vi "Baud rate Detect1.vi"(10 "DevIndex":u32, 11 "type":u16(ring)=2 items=["USB-CAN"=2, "USB-CAN2.0"=3]) -> ()   [LabVIEW 2011]
uses:
  _USB_CAN_GLOBAL_.vi
  data/VCI_CAN.dll
panel:
  in  "cancel":bool
  in  "ok":bool
  out "br":u32(ring)=8 caption="当前波特率:" items=["5k bps"=1, "10k bps"=2, "20k bps"=3, "40k bps"=4, "50k bps"=5, "80k bps"=6, "100k bps"=7, "125k bps"=8, "200k bps"=9, "250k bps"=10, "400k bps"=11, "500k bps"=12, "666k bps"=13, "800k bps"=14, "1000k bps"=15, "self define"=16]
  out "chl":u32 caption="正在侦测：" format="通道%d"
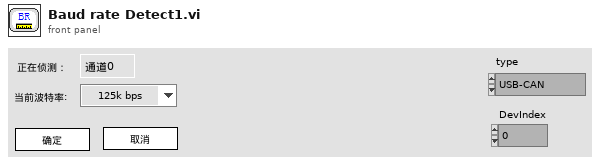
[diagram p1: front panel]
types:
  T1 = cluster{"AccCode":u32, "AccMask":u32, "Reserved":u32, "Filter":u8, "kCanBaud":u8, "Timing0":u8, "Timing1":u8, "Mode":u8}
  T2 = enum8{"Enabled", "Disabled", "Disabled and Grayed Out"}
  T3 = cluster{"ErrInterrupt":u8, "regMode":u8, "regStatus":u8, "regALCapture":u8, "regECCapture":u8, "regEWLimit":u8, "regRECounter":u8, "regTECounter":u8, "Reserved":u32}
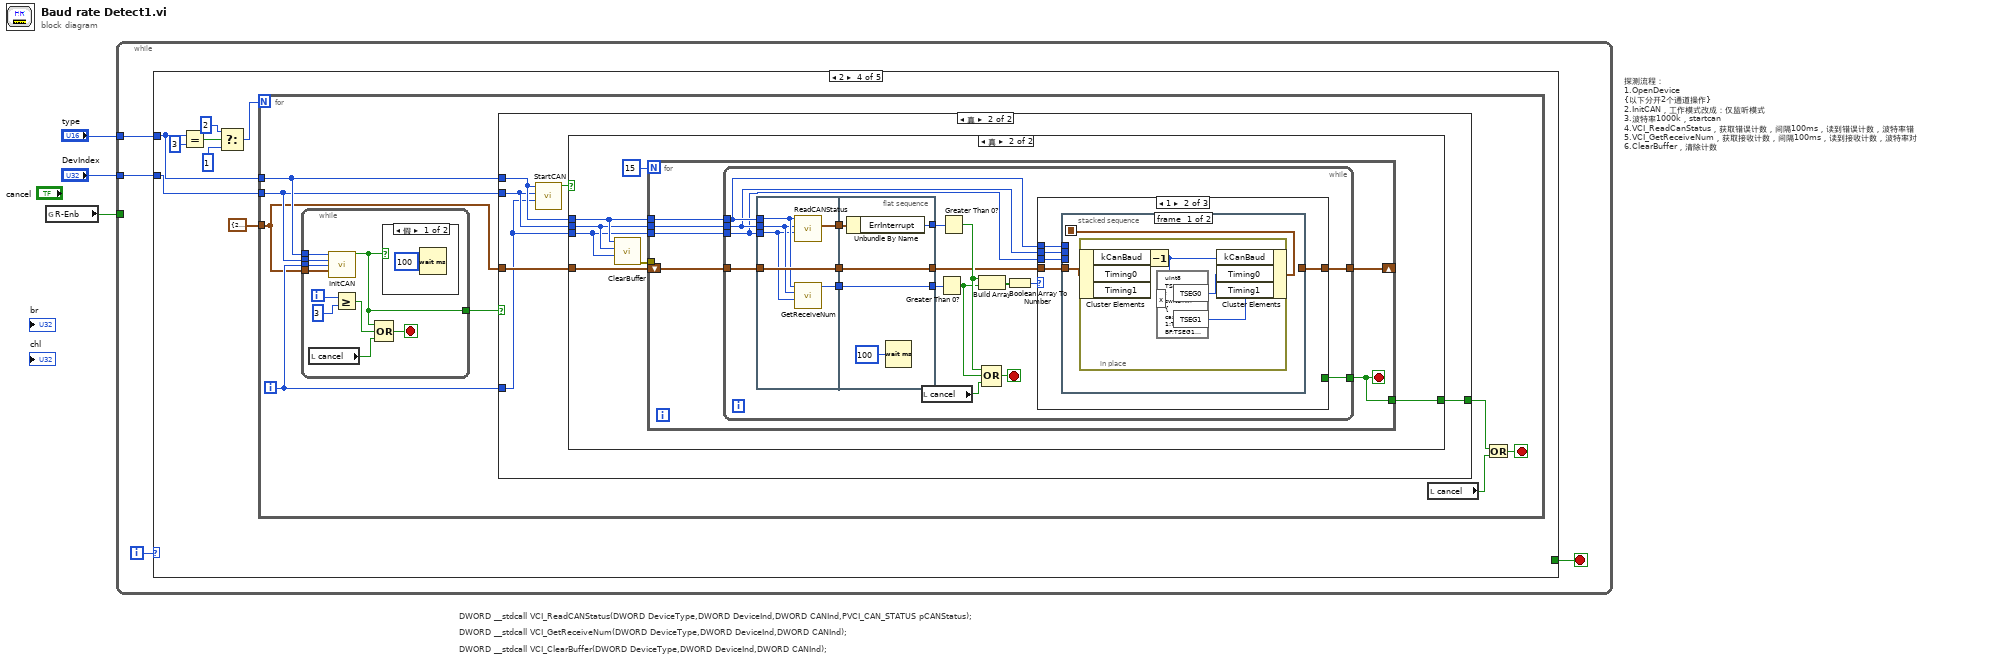
[diagram p0: block diagram]
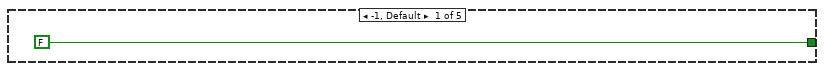
[diagram p2: hidden frame]
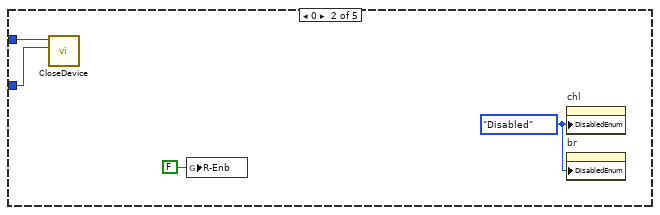
[diagram p3: hidden frame]
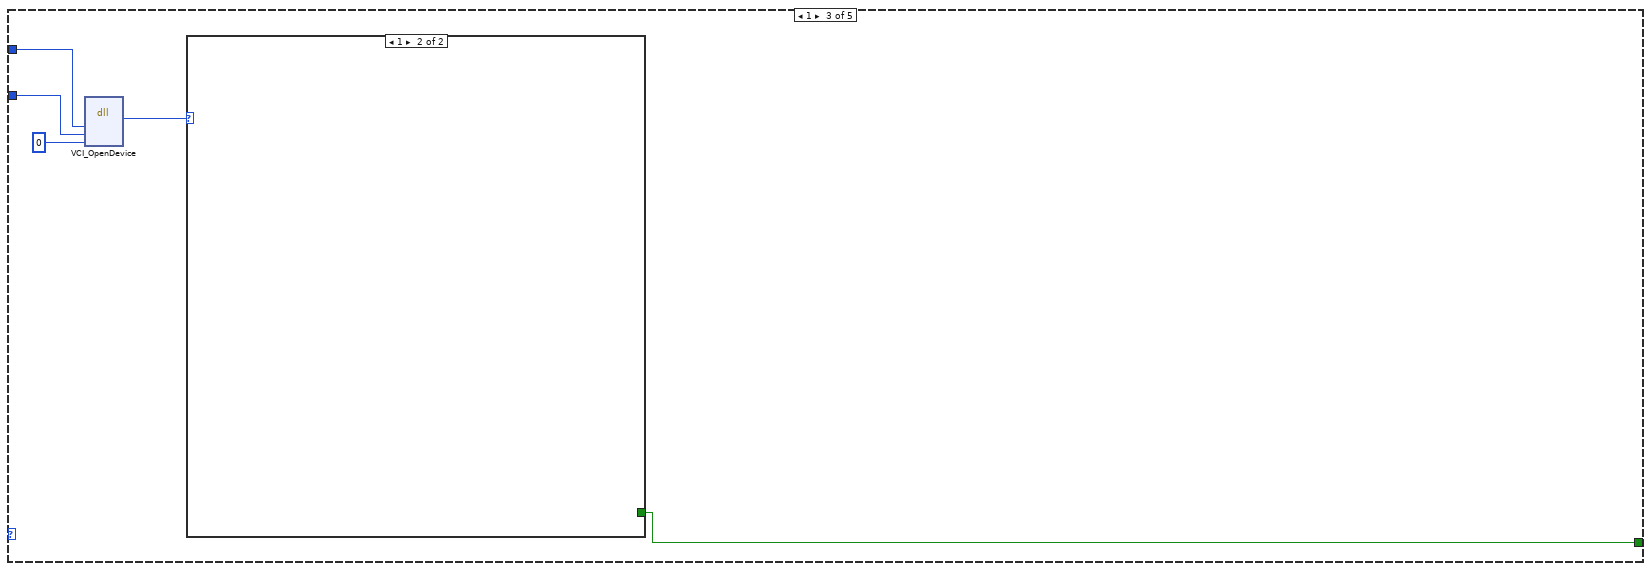
[diagram p4: hidden frame]
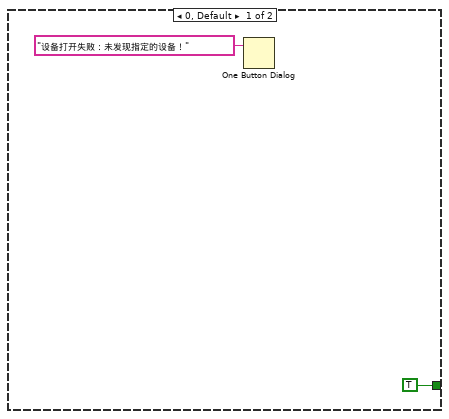
[diagram p5: hidden frame]
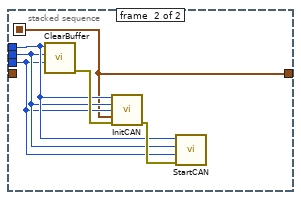
[diagram p9: hidden frame]
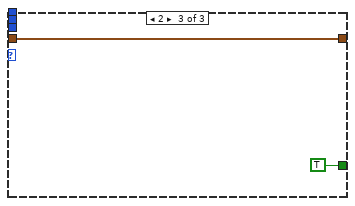
[diagram p10: hidden frame]
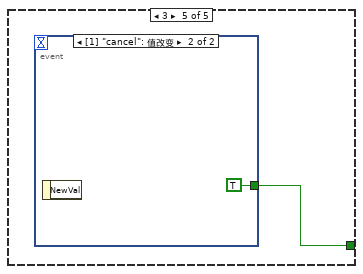
[diagram p12: hidden frame]
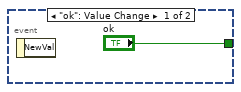
[diagram p13: hidden frame]
diagram:
  # "DWORD __stdcall VCI_ClearBuffer(DWORD DeviceType,DWORD DeviceInd,DWORD CANInd);"
  # "DWORD __stdcall VCI_GetReceiveNum(DWORD DeviceType,DWORD DeviceInd,DWORD CANInd);"
  # "DWORD __stdcall VCI_ReadCANStatus(DWORD DeviceType,DWORD DeviceInd,DWORD CANInd,PVCI_CAN_STATUS pCANStatus);"
  # "探测流程：\n1.OpenDevice\n{以下分开2个通道操作}\n2.InitCAN，工作模式改成：仅监听模式\n3.波特率1000k，startcan\n4.VCI_ReadCanStatus，获取错误计数，间隔100ms，读到错误计数，波特率错\n5.VCI_GetReceiveNum，获取接收计数，间隔100ms，读到接收计数，波特率对\n6.ClearBuffer，清除计数"
  n1 = global read "_USB_CAN_GLOBAL_.vi" "R-Enb"() -> (w3:bool)
  n2 = while {
    tunnel: w3 -> [_]
    tunnel: "type" -> [w5]
    tunnel: "DevIndex" -> [w4]
    i -> [w7]
    stop <- w6 stop-if-true
    n3 = case shown="2" w7 {
      tunnel: [FALSE _ w13 _ w115] -> w6
      tunnel: w5 -> [_ w11 w17 w22 _]
      tunnel: w4 -> [_ w10 w16 w21 _]
      frame -1, Default {
      }
      frame 0 {
        w9 = T2."Disabled" ("禁用")
        n4 = call "CloseDevice.vi"("DeviceInd"=w10, "type"=w11) -> ()  [unwired: 8 in, 2 out]
        n5 = global write "_USB_CAN_GLOBAL_.vi" "R-Enb"(FALSE ("R-Enb")) -> ()
        n6 = property on="chl" class="DigNum (严格)"("DisabledEnum"=w9) -> ()  [unwired: 2 in, 2 out]
        n7 = property on="br" class="Ring (严格)"("DisabledEnum"=w9) -> ()  [unwired: 2 in, 2 out]
      }
      frame 1 {
        n8 = dll-call lib="PTH1Kabs D\t董海成\t上位机2.进行中USB-CAN TooldataVCI_CAN.dll" fn="VCI_OpenDevice"("DevType"=w17, "DevIndex"=w16, "Reserved"=u32 0) -> ("返回类型"=w14:u32)  [unwired: 6 in, 2 out]
        n9 = case shown="1" w14 {
          tunnel: [TRUE _] -> w13
          frame 0, Default {
            n10 = One Button Dialog(message="设备打开失败：未发现指定的设备！" ("消息")) -> ()  [unwired: 1 in, 1 out]
          }
          frame 1 {
          }
        }
      }
      frame 2 {
        n11 = Equal?(x=w22, y=u16 3) -> (x = y?=w26:bool)
        n12 = Select(t=2, s=w26, f=1) -> (s? t:f=w23:i32)
        n13 = for {
          N: w23 -> [_]
          tunnel: w22 -> [w34]
          tunnel: w21 -> [w33]
          tunnel: T1 {"AccCode"=2147483648, "AccMask"=4294967295, "Reserved"=0, "Filter"=0, "kCanBaud"=15, "Timing0"=0, "Timing1"=20, "Mode"=2} ("pInitConfig") -> [w31]
          i -> [w32]
          stop <- w28 stop-if-true
          n14 = while {
            tunnel: w34 -> [w113]
            tunnel: w33 -> [w112]
            tunnel: w32 -> [w111]
            tunnel: w31 -> [w110]
            tunnel: [w105] -> w35
            i -> [w109]
            stop <- w106 stop-if-true
            n15 = local read "cancel"() -> (w104:bool)
            n16 = call "InitCAN.vi"("DeviceType"=w113, "DeviceInd"=w112, "CANInd"=w111, "pInitConfig"=w110) -> ("Success"=w105:bool)  [unwired: 10 in, 1 out]
            n17 = Greater Or Equal?(x=w109, y=3) -> (x >= y?=w107:bool)
            n18 = Compound Arithmetic op=OR(w105, w107, w104) -> (w106:bool)
            n19 = case shown="假" w105 {
              frame False {
                n20 = Wait (ms)(milliseconds to wait=u32 100 ("等待时间（毫秒）")) -> ()  [unwired: 1 out]
              }
              frame True {
              }
            }
          }
          n21 = case shown="真" w35 {
            tunnel: w34 -> [_ w39]
            tunnel: w33 -> [_ w38]
            tunnel: w32 -> [_ w37]
            tunnel: w31 -> [_ w40]
            tunnel: [_ w36] -> w30
            frame False {
            }
            frame True {
              n22 = call "StartCAN.vi"("CANInd"=w37, "DeciceInd"=w38, "DeviceType"=w39) -> ("Valid"=w41:bool)  [unwired: 7 in, 1 out]
              n23 = case shown="真" w41 {
                tunnel: w40 -> [_ w47]
                tunnel: w39 -> [_ w46]
                tunnel: w38 -> [_ w45]
                tunnel: w37 -> [_ w44]
                tunnel: [_ w42] -> w36
                frame False {
                }
                frame True {
                  n24 = call "ClearBuffer.vi"("CANInd"=w44, "DeciceInd"=w45, "DeviceType"=w46) -> ("error out"=w43:errorcluster)  [unwired: 7 in, 1 out]
                  n25 = for {
                    N: 15 -> [_]
                    shift-right: [w50] -> _
                    shift-left: w47 -> [w51]
                    tunnel: w46 -> [w54]
                    tunnel: w45 -> [w53]
                    tunnel: w44 -> [w52]
                    tunnel: w43 -> [_]
                    tunnel: [w49] -> w42
                    stop <- w49 stop-if-true
                    n26 = while {
                      tunnel: w54 -> [w58]
                      tunnel: w53 -> [w57]
                      tunnel: w52 -> [w56]
                      tunnel: w51 -> [w69]
                      tunnel: [w59] -> w50
                      tunnel: [w55] -> w49
                      stop <- w65 stop-if-true
                      n27 = flat-sequence {
                        tunnel: w58 -> [w96]
                        tunnel: w57 -> [w95]
                        tunnel: w56 -> [w94]
                        tunnel: [w98] -> w72
                        tunnel: w69 -> [w97]
                        tunnel: [w97] -> w71
                        tunnel: [w93] -> w70
                        tunnel: w72 -> [w102]
                        tunnel: w71 -> [w100]
                        tunnel: w70 -> [w99]
                        tunnel: [w101] -> w68
                        tunnel: [w100] -> w60
                        tunnel: [w99] -> w67
                        frame #0 {
                          n28 = call "ReadCANStatus.vi"("CANInd"=w94, "DeciceInd"=w95, "DeviceType"=w96) -> ("VCI_CAN_STATUS"=w98:T3)  [unwired: 6 in, 2 out]
                          n29 = call "GetReceiveNum.vi"("CANInd"=w94, "DeciceInd"=w95, "DeviceType"=w96) -> ("FrmsUnRead"=w93:u32)  [unwired: 7 in, 1 out]
                        }
                        frame #1 {
                          n30 = Unbundle By Name(w102) -> ("ErrInterrupt"=w101:u8)
                          n31 = Wait (ms)(milliseconds to wait=u32 100 ("等待时间（毫秒）")) -> ()  [unwired: 1 out]
                        }
                      }
                      n32 = local read "cancel"() -> (w66:bool)
                      n33 = Greater Than 0?(x=w67) -> (x > 0?=w63:bool)
                      n34 = Greater Than 0?(x=w68) -> (x > 0?=w64:bool)
                      n35 = Build Array(w64, w63) -> (w62:bool[])
                      n36 = Compound Arithmetic op=OR(w64, w63, w66) -> (w65:bool)
                      n37 = Boolean Array To Number(Boolean array=w62) -> (number=w61:u32)
                      n38 = case shown="1" w61 {
                        tunnel: w60 -> [w73 w78 w92]
                        tunnel: [w73 w74 w92] -> w59
                        tunnel: w58 -> [_ w77 _]
                        tunnel: w57 -> [_ w76 _]
                        tunnel: w56 -> [_ w75 _]
                        tunnel: [_ _ TRUE] -> w55
                        frame 0, Default {
                        }
                        frame 1 {
                          n39 = stacked-sequence {
                            seq-local: [w79 _] -> [_ w85]
                            tunnel: w78 -> [w80 _]
                            tunnel: w77 -> [_ w88]
                            tunnel: w76 -> [_ w87]
                            tunnel: w75 -> [_ w86]
                            tunnel: [_ w85] -> w74
                            frame #0 {
                              n40 = in-place {
                                n41 = in-place-cluster #1(w80) -> ("kCanBaud"=w84:u8)  [unwired: 2 out]
                                n42 = Decrement(x=w84) -> (x-1=w83:u8)
                                n43 = formula code="uInt8 TSEG0,TSEG1;\nswitch(x)\n{ \ncase 1:TSEG0=0xBF;TSEG1=0xFF;break;\ncase 2:TSEG0=0x31;TSEG1=0x1c;break;\ncase 3:TSEG0=0x18;TSEG1=0x1c;break;\ncase 4:TSEG0=0x87;TSEG1=0xff;break;\ncase 5:TSEG0=0x09;TSEG1=0x1c;break;\ncase 6:TSEG0=0x83;TSEG1=0xff;break;\ncase 7:TSEG0=0x04;TSEG1=0x1c;break;\ncase 8:TSEG0=0x03;TSEG1=0x1c;break;\ncase 9:TSEG0=0x81;TSEG1=0xfa;break;\ncase 10:TSEG0=0x01;TSEG1=0x1c;break;\ncase 11:TSEG0=0x80;TSEG1=0xfa;break;\ncase 12:TSEG0=0x00;TSEG1=0x1c;break;\ncase 13:TSEG0=0x80;TSEG1=0xb6;break;\ncase 14:TSEG0=0x00;TSEG1=0x16;break;\ncase 15:TSEG0=0x00;TSEG1=0x14;break;\ndefault:TSEG0=0x00;TSEG1=0x00;\n}"("x"=w83) -> ("TSEG0"=w82:u8, "TSEG1"=w81:u8)
                                n44 = in-place-cluster #1("kCanBaud"=w83, "Timing0"=w82, "Timing1"=w81) -> (w79:T1)
                              }
                            }
                            frame #1 {
                              n45 = call "ClearBuffer.vi"("CANInd"=w86, "DeciceInd"=w87, "DeviceType"=w88) -> ("error out"=w90:errorcluster)  [unwired: 7 in, 1 out]
                              n46 = call "InitCAN.vi"("DeviceType"=w88, "DeviceInd"=w87, "CANInd"=w86, "pInitConfig"=w85, "error in (no error)"=w90) -> ("error out"=w89:errorcluster)  [unwired: 9 in, 1 out]
                              n47 = call "StartCAN.vi"("error in (no error)"=w89, "CANInd"=w86, "DeciceInd"=w87, "DeviceType"=w88) -> ()  [unwired: 6 in, 2 out]
                            }
                          }
                        }
                        frame 2 {
                        }
                      }
                    }
                  }
                }
              }
            }
          }
          n48 = local read "cancel"() -> (w29:bool)
          n49 = Or(x=w30, y=w29) -> (x .or. y?=w28:bool)
        }
      }
      frame 3 {
        n50 = event shown="[1] \"cancel\": 值改变" {
          selector: _ -> [_ _]
          dyn-events: _ -> [_ _]
          timeout: _ -> [_ _]
          tunnel: ["ok" TRUE ("ok")] -> w115
          event "ok": Value Change {
            n51 = event-data() -> ()  [unwired: 1 in, 1 out]
          }
          event "cancel": Value Change {
            n52 = event-data() -> ()  [unwired: 1 in, 1 out]
          }
        }
      }
    }
  }
